vi "EightTimer.vi"() -> ()   [LabVIEW 2015]
uses:
  <vilib>/Platform/TimedLoop/XDataNode/timing_clust.ctl
  <vilib>/Platform/TimedLoop/XDataNode/nitl_modes.ctl
  <vilib>/Platform/TimedLoop/XDataNode/wakeup.ctl
  <vilib>/rvi/Emulation/niFpgaSctlEmulationGetInTimedLoop.vi
  <vilib>/rvi/Emulation/niFpgaEmulationReportErrorSimple.vi
  <vilib>/rvi/Emulation/niFpgaGetClockAttributes.vi
  <vilib>/rvi/Emulation/niFpgaCriticalErrorInLSC.vi
  TickTocks/Tock7.vi
  TickTocks/Tick7.vi
  TickTocks/Tock6.vi
  TickTocks/Tick6.vi
  TickTocks/Tock5.vi
  TickTocks/Tick5.vi
  TickTocks/Tock4.vi
  TickTocks/Tick4.vi
  TickTocks/Tock3.vi
  TickTocks/Tick3.vi
  TickTocks/Tock2.vi
  TickTocks/Tick2.vi
  TickTocks/Tock1.vi
  TickTocks/Tick1.vi
  TickTocks/Tock0.vi
  TickTocks/Tick0.vi
  <vilib>/platform/TimedLoop/XDataNode/XDataNode.xnode
  <vilib>/Platform/TimedLoop/XDataNode/XDNodeRunTimeDep.lvlib
  Timers.lvlib
panel:
  out "MaxTimes":u32[](array[numeric])
  out "Times":u32[](array[numeric])
  in  "resetMaxTime":bool
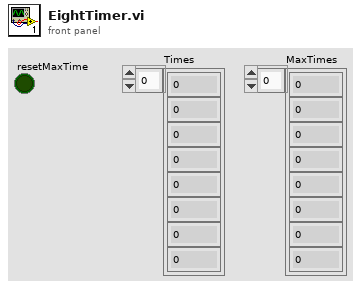
[diagram p1: front panel]
types:
  T1 = typedef "Timers.lvlib/TimerRegisters.ctl" = cluster{"Tick0":refnum<k21>, "Tock0":refnum<k21>, "Tick1":refnum<k21>, "Tock1":refnum<k21>, "Tick2":refnum<k21>, "Tock2":refnum<k21>, "Tick3":refnum<k21>, "Tock3":refnum<k21>, "Tick4":refnum<k21>, "Tock4":refnum<k21>, "Tick5":refnum<k21>, "Tock5":refnum<k21>, "Tick6":refnum<k21>, "Tock6":refnum<k21>, "Tick7":refnum<k21>, "Tock7":refnum<k21>}
  T2 = typedef "XDNodeRunTimeDep.lvlib/timing_clust.ctl" = cluster{"Expected End [f-1]":u64, "Actual End [f-1]":u64, "Finished Late? [f-1]":bool, "Expected End [i-1]":u64, "Actual End [i-1]":u64, "Finished Late? [i-1]":bool, "Expected Start [i]":u64, "Actual Start [i]":u64, "Expected Start [f]":u64, "Actual Start [f]":u64, "Source Name":string, "Structure Name":string, "Period":i64, "Deadline":i64, "Offset":i64, "Start":i64, "Priority":i32, "Timeout":i32, "Mode":T3, "Wakeup Reason":T4, "Error":errorcluster, "Source Type":string, "Secondary Source Type":string, "Global End Time":u64, "Global Start Time":u64, "Frame Duration":u64, "Iteration Duration":u64, "Assigned CPU":i32, "I/O Scan Engine Mode":u32}
  T3 = typedef "XDNodeRunTimeDep.lvlib/nitl_modes.ctl" = enum32{"No Change", "Process missed periods, maintain original phase", "Discard missed periods, maintain original phase", "Process missed periods, ignore original phase", "Discard missed periods, ignore original phase"}
  T4 = typedef "XDNodeRunTimeDep.lvlib/wakeup.ctl" = enum32{"Normal", "Aborted", "Asynchronous wakeup", "Timing source error", "Timed loop error", "Timeout"}
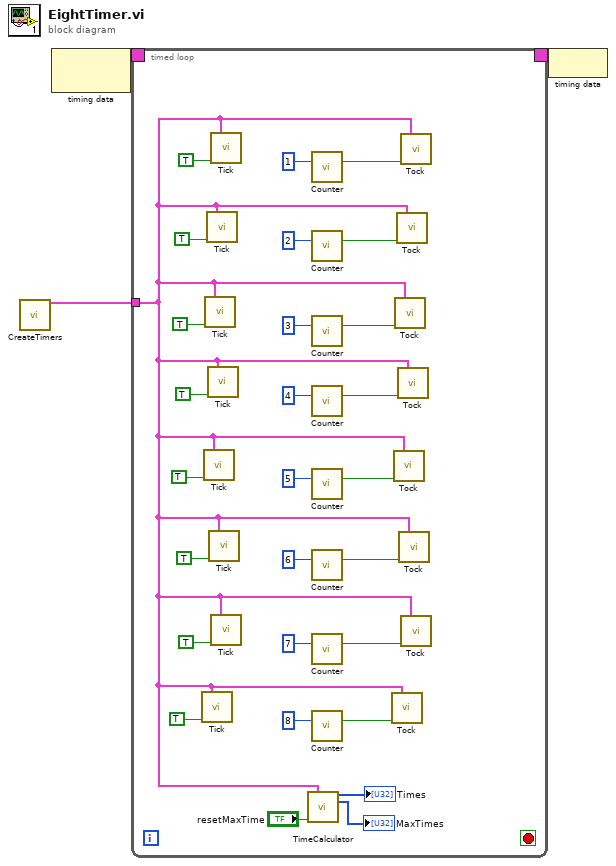
[diagram p0: block diagram]
diagram:
  n1 = call "CreateTimers.vi"() -> ("TimerRegisters"=w1:T1)  [unwired: 15 in]
  n2 = node-c288() -> (w3:T2)  [unwired: 1 in]
  n3 = timed-loop {
    timing: w3 -> [_]
    timing-out: [_] -> w2
    tunnel: w1 -> [w7]
    stop <- _ stop-if-true
    n4 = call-poly "Tick.vi"("TimerRegisters"=w7, "valid input"=TRUE) -> ()  [unwired: 13 in, 1 out]
    n5 = call-poly "Tick.vi"("TimerRegisters"=w7, "valid input"=TRUE) -> ()  [unwired: 13 in, 1 out]
    n6 = call-poly "Tick.vi"("TimerRegisters"=w7, "valid input"=TRUE) -> ()  [unwired: 13 in, 1 out]
    n7 = call-poly "Tick.vi"("TimerRegisters"=w7, "valid input"=TRUE) -> ()  [unwired: 13 in, 1 out]
    n8 = call-poly "Tick.vi"("TimerRegisters"=w7, "valid input"=TRUE) -> ()  [unwired: 13 in, 1 out]
    n9 = call-poly "Tick.vi"("TimerRegisters"=w7, "valid input"=TRUE) -> ()  [unwired: 13 in, 1 out]
    n10 = call-poly "Tick.vi"("TimerRegisters"=w7, "valid input"=TRUE) -> ()  [unwired: 13 in, 1 out]
    n11 = call-poly "Tick.vi"("TimerRegisters"=w7, "valid input"=TRUE) -> ()  [unwired: 13 in, 1 out]
    n12 = call "TimeCalculator.vi"("TimerRegisters"=w7, "resetMaxTime"="resetMaxTime") -> ("Times"=→"Times":u32[], "MaxTimes"=→"MaxTimes":u32[])  [unwired: 12 in]
    n13 = call "Counter.vi"("ticks"=u16 1) -> ("ding"=w30:bool)  [unwired: 14 in]
    n14 = call "Counter.vi"("ticks"=u16 2) -> ("ding"=w27:bool)  [unwired: 14 in]
    n15 = call "Counter.vi"("ticks"=u16 3) -> ("ding"=w24:bool)  [unwired: 14 in]
    n16 = call "Counter.vi"("ticks"=u16 4) -> ("ding"=w21:bool)  [unwired: 14 in]
    n17 = call "Counter.vi"("ticks"=u16 5) -> ("ding"=w18:bool)  [unwired: 14 in]
    n18 = call "Counter.vi"("ticks"=u16 6) -> ("ding"=w15:bool)  [unwired: 14 in]
    n19 = call "Counter.vi"("ticks"=u16 7) -> ("ding"=w12:bool)  [unwired: 14 in]
    n20 = call "Counter.vi"("ticks"=u16 8) -> ("ding"=w9:bool)  [unwired: 14 in]
    n21 = call-poly "Tock.vi"("TimerRegisters"=w7, "valid input"=w9) -> ()  [unwired: 13 in, 1 out]
    n22 = call-poly "Tock.vi"("TimerRegisters"=w7, "valid input"=w18) -> ()  [unwired: 13 in, 1 out]
    n23 = call-poly "Tock.vi"("TimerRegisters"=w7, "valid input"=w24) -> ()  [unwired: 13 in, 1 out]
    n24 = call-poly "Tock.vi"("TimerRegisters"=w7, "valid input"=w27) -> ()  [unwired: 13 in, 1 out]
    n25 = call-poly "Tock.vi"("TimerRegisters"=w7, "valid input"=w21) -> ()  [unwired: 13 in, 1 out]
    n26 = call-poly "Tock.vi"("TimerRegisters"=w7, "valid input"=w15) -> ()  [unwired: 13 in, 1 out]
    n27 = call-poly "Tock.vi"("TimerRegisters"=w7, "valid input"=w30) -> ()  [unwired: 13 in, 1 out]
    n28 = call-poly "Tock.vi"("TimerRegisters"=w7, "valid input"=w12) -> ()  [unwired: 13 in, 1 out]
  }
  n29 = node-c288(w2) -> ()
